vi "Query Multi Eval Meas State.vi"(8 "error in (no error)":errorcluster, 9 "Instance (1)":T1=1, 11 "VISA resource name":refnum<visa-resource-name>) -> (0 "error out":errorcluster, 1 "Sync State":i32, 2 "Main State":i32, 3 "VISA resource name out":refnum<visa-resource-name>, 4 "Resources State":i32)   [LabVIEW 2020, in "Rohde&Schwarz CMWXP NR FR1 Measurement.lvlib"]
doc: "Queries the main measurement state and the measurement substates. Both measurement substates are relevant for running measurements only. Use FETCh:...:STATe? to query the main measurement state only. Use INITiate..., STOP..., ABORt... to change the measurement state.\n\nAttribute:\nRSCMWXPNRFR1M_ATTR_MULTI_EVAL_MEAS_MEASUREMENT_STATE\n\nRemote-control command:\nFETCh:NRSub:MEAS<i>:MEValuation:STATe:ALL?"
uses:
  <instrlib>/Rohde&Schwarz CMWXP NR FR1 Measurement/Rohde&Schwarz CMWXP NR FR1 Measurement.lvlib
  <instrlib>/Rohde&Schwarz CMWXP NR FR1 Measurement/Private/_Instance.ctl
  <instrlib>/Rohde&Schwarz CMWXP NR FR1 Measurement/Private/rsidr_core.llb/rsidr_core.lvlib
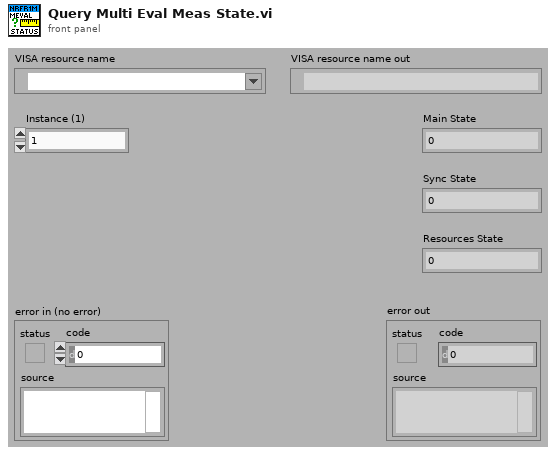
[diagram p1: front panel]
types:
  T1 = typedef "Rohde&Schwarz CMWXP NR FR1 Measurement.lvlib/_Instance.ctl" = i32
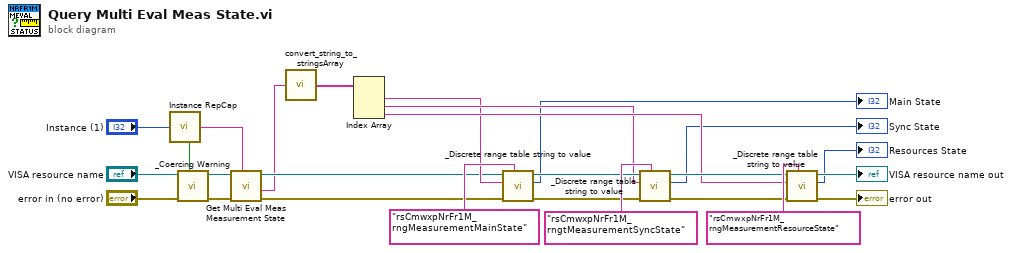
[diagram p0: block diagram]
diagram:
  n1 = call <instrlib>:"Instance RepCap.vi"("Instance In"="Instance (1)") -> ("In Range?"=w26:bool, "RepCap Identifier Out"=w2:string)  [unwired: 1 in]
  n2 = call <instrlib>:"_Coercing Warning.vi"("In Range?"=w26, "error in (no error)"="error in (no error)", "VISA resource name"="VISA resource name") -> ("error out"=w6:errorcluster, "VISA resource name out"=w5:refnum<visa-resource-name>)  [unwired: 7 in]
  n3 = call "Get Multi Eval Meas Measurement State"("Repeated Capabilities"=w2, "error in (no error)"=w6, "instrument handle"=w5) -> ("error out"=w4:errorcluster, "Multi Eval Meas Measurement State"=w1:string, "instrument handle out"=w3:refnum<visa-resource-name>)  [unwired: 6 in]
  n4 = call <instrlib>:"convert_string_to_stringsArray.vi"("String in"=w1) -> ("string array out"=w24:string[])  [unwired: 3 in, 1 out]
  n5 = Index Array(array=w24) -> (element #1=w15:string, element #2=w16:string, element #3=w17:string)  [unwired: 3 in]
  n6 = call <instrlib>:"_Discrete range table string to value.vi"("Discrete Range Table Identifier"="rsCmwxpNrFr1M_rngMeasurementMainState", "error in (no error)"=w4, "String Value In"=w15, "VISA resource name"=w3) -> ("error out"=w22:errorcluster, "Enum Value"=→"Main State":i32, "VISA resource name out"=w18:refnum<visa-resource-name>)  [unwired: 5 in]
  n7 = call <instrlib>:"_Discrete range table string to value.vi"("Discrete Range Table Identifier"="rsCmwxpNrFr1M_rngtMeasurementSyncState", "error in (no error)"=w22, "String Value In"=w16, "VISA resource name"=w18) -> ("error out"=w20:errorcluster, "Enum Value"=→"Sync State":i32, "VISA resource name out"=w19:refnum<visa-resource-name>)  [unwired: 5 in]
  n8 = call <instrlib>:"_Discrete range table string to value.vi"("Discrete Range Table Identifier"="rsCmwxpNrFr1M_rngMeasurementResourceState", "error in (no error)"=w20, "String Value In"=w17, "VISA resource name"=w19) -> ("error out"=→"error out":errorcluster, "Enum Value"=→"Resources State":i32, "VISA resource name out"=→"VISA resource name out":refnum<visa-resource-name>)  [unwired: 5 in]
